vi "sys_integration.vi"() -> ()   [LabVIEW 2016, in "Utilities.lvlib" / "_TEST.lvlib"]
uses:
  _TEST.lvlib
  Drivers/C8855-01/Trigger Mode.ctl
  Drivers/C8855-01/Transfer Mode.ctl
  <vilib>/DAQmx/write.llb/DAQmx Write (Analog 1D DBL 1Chan NSamp).vi
  <vilib>/DAQmx/read.llb/DAQmx Read (Analog 1D DBL 1Chan NSamp).vi
  <vilib>/DAQmx/create/channels.llb/DAQmx Create Channel (AO-Voltage-Basic).vi
  <vilib>/DAQmx/create/channels.llb/DAQmx Create Channel (AI-Voltage-Basic).vi
  <vilib>/DAQmx/create/channels.llb/DAQmx Create Channel (CO-Pulse Generation-Time).vi
  <vilib>/DAQmx/configure/timing.llb/DAQmx Timing (Implicit).vi
  <vilib>/DAQmx/configure/timing.llb/DAQmx Timing (Sample Clock).vi
  <vilib>/DAQmx/configure/trigger.llb/DAQmx Start Trigger (Digital Edge).vi
  <vilib>/DAQmx/miscellaneous.llb/DAQmx Fill In Error Info.vi
  Drivers/C8855-01/C8855-01.lvlib
  <vilib>/measure/NI_MABase.lvlib
  <resource>/objmgr/daqmx.rc
panel:
  in  "Repeats":u16=100
  in  "Offset (V)":dbl format="%0.2p"
  out "Actual Galvo Freq (Hz)":dbl
  in  "Amplitude (V)":dbl=1.0 format="%#_13g"
  out "Sampling Freq (Hz)":dbl
  out "# / Period":i32
  out "Gate Time (s)":dbl
  in  "Galvo Freq (Hz)":u32=100
  in  "Gate Time (us)":u32=100
  out "Data":cluster{dbl[], u16[]}(graph)
  out "Photon Counter ID":u8
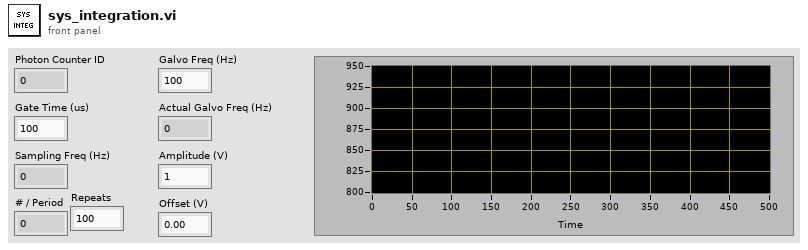
[diagram p1: front panel]
types:
  T1 = typedef "Drivers.lvlib/C8855-01.lvlib/Transfer Mode.ctl" = u8
  T2 = typedef "Drivers.lvlib/C8855-01.lvlib/Trigger Mode.ctl" = u8
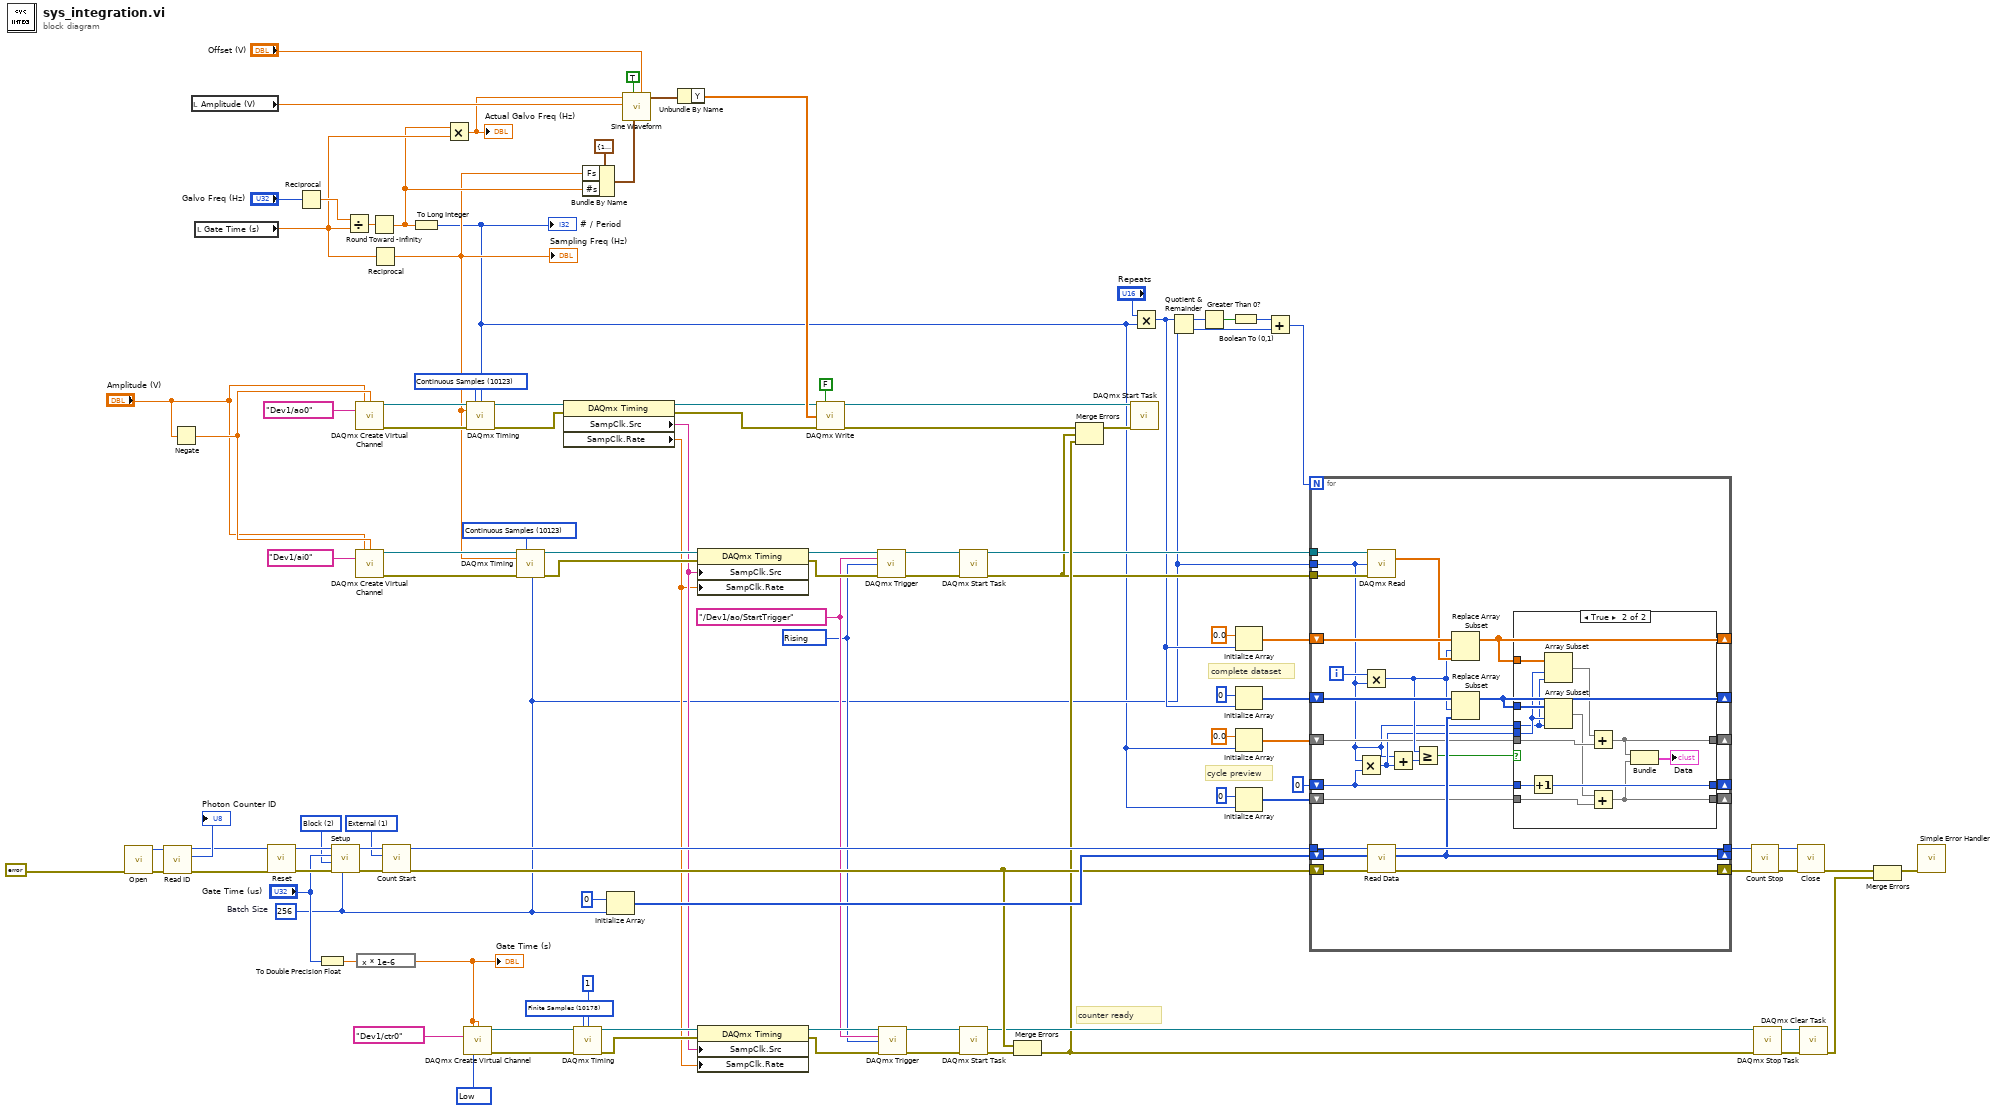
[diagram p0: block diagram]
diagram:
  w32 = 10214 items=["High"=10192, "Low"=10214] ("idle state")
  w28 = 10280 items=["Rising"=10280, "Falling"=10171] ("edge")
  w29 = tag "/Dev1/ao/StartTrigger" ("source")
  w43 = 10123 items=["Finite Samples"=10178, "Continuous Samples"=10123, "Hardware Timed Single Point"=12522] ("sample mode")
  w64 = 10123 items=["Finite Samples"=10178, "Continuous Samples"=10123, "Hardware Timed Single Point"=12522] ("sample mode")
  w78 = T1 2 items=["Single"=1, "Block"=2] ("Transfer Mode")
  w83 = 10178 items=["Finite Samples"=10178, "Continuous Samples"=10123, "Hardware Timed Single Point"=12522] ("sample mode")
  w10 = 256  # Batch Size
  w95 = T2 1 items=["Software", "External"] ("Trigger Mode")
  # "cycle preview"
  # "complete dataset"
  # "counter ready"
  n1 = call "Open.vi"("error in (no error)"=errorcluster {"status"=FALSE, "code"=0, "source"=""}) -> ("error out"=w103:errorcluster, "Handle"=w104:u32)  [unwired: 9 in]
  n2 = call "Read ID.vi"("error in (no error)"=w103, "handle in"=w104) -> ("error out"=w101:errorcluster, "ID"=→"Photon Counter ID":u8, "handle out"=w100:u32)  [unwired: 7 in]
  n3 = Negate(x="Amplitude (V)") -> (-x=w63:dbl)
  n4 = local read "Amplitude (V)"() -> (w59:dbl)
  n5 = local read "Gate Time (s)"() -> (w58:dbl)
  n6 = call "Reset.vi"("error in (no error)"=w101, "handle in"=w100) -> ("error out"=w99:errorcluster, "handle out"=w96:u32)  [unwired: 8 in]
  n7 = Reciprocal(x="Galvo Freq (Hz)") -> (1/x=w67:dbl)
  n8 = To Double Precision Float(number="Gate Time (us)") -> (double precision float=w86:dbl)
  n9 = call "Setup.vi"("Number of Gate"=w10, "error in (no error)"=w99, "Transfer Mode"=w78, "Gate Time (us)"="Gate Time (us)", "Handle"=w96) -> ("error out"=w98:errorcluster, "Handle out"=w97:u32)  [unwired: 5 in]
  n10 = Divide(x=w67, y=w58) -> (x/y=w65:dbl)
  n11 = call-poly <vilib>:"DAQmx Create Virtual Channel.vi"("maximum value"="Amplitude (V)", "minimum value"=w63, "physical channels"=tag "Dev1/ao0") -> ("task out"=w70:refnum<k21>, "error out"=w69:errorcluster)  [unwired: 11 in]
  n12 = call-poly <vilib>:"DAQmx Create Virtual Channel.vi"("maximum value"="Amplitude (V)", "minimum value"=w63, "physical channels"=tag "Dev1/ai0") -> ("task out"=w46:refnum<k21>, "error out"=w45:errorcluster)  [unwired: 11 in]
  n13 = expression code="x * 1e-6"(w86) -> (w66:dbl)
  "Gate Time (s)" <- w66
  n14 = Round Toward -Infinity(1:w65) -> (0:w56:dbl)
  n15 = Reciprocal(x=w58) -> (1/x=w44:dbl)
  "Sampling Freq (Hz)" <- w44
  n16 = call "Count Start.vi"("error in (no error)"=w98, "Trigger Mode"=w95, "handle in"=w97) -> ("error out"=w74:errorcluster, "handle out"=w93:u32)  [unwired: 7 in]
  n17 = To Long Integer(number=w56) -> (32bit integer=w4:i32)
  "# / Period" <- w4
  n18 = Multiply(x=w56, y=w58) -> (x*y=w57:dbl)
  "Actual Galvo Freq (Hz)" <- w57
  n19 = call-poly <vilib>:"DAQmx Create Virtual Channel.vi"("high time"=w66, "low time"=w66, "counter"=tag "Dev1/ctr0" ("physical channels"), "idle state"=w32) -> ("task out"=w85:refnum<k21>, "error out"=w84:errorcluster)  [unwired: 10 in]
  n20 = call-poly <vilib>:"DAQmx Timing.vi"("task/channels in"=w70, "sample mode"=w64, "samples per channel"=w4, "rate"=w44, "error in"=w69) -> ("task out"=w53:refnum<k21>, "error out"=w48:errorcluster)  [unwired: 9 in]
  n21 = call-poly <vilib>:"DAQmx Timing.vi"("task/channels in"=w46, "sample mode"=w43, "samples per channel"=w10, "rate"=w44, "error in"=w45) -> ("task out"=w42:refnum<k21>, "error out"=w40:errorcluster)  [unwired: 9 in]
  n22 = property class="DAQmx Timing"(reference=w53, error in=w48) -> (reference out=w49:refnum<k21>, error out=w47:errorcluster, "SampClk.Src"=w34:tag, "SampClk.Rate"=w33:dbl)
  n23 = call-poly <vilib>:"DAQmx Timing.vi"("task/channels in"=w85, "sample mode"=w83, "samples per channel"=1, "error in"=w84) -> ("task out"=w82:refnum<k21>, "error out"=w35:errorcluster)  [unwired: 10 in]
  n24 = Bundle By Name(cluster=cluster{"Fs":dbl, "#s":dbl} {"Fs"=1000.0, "#s"=1000.0} ("sampling info"), "Fs"=w44, "#s"=w56) -> (w60:cluster{"Fs":dbl, "#s":dbl})
  n25 = Initialize Array(u16 0 ("element"), w10) -> (w92:u16[])
  n26 = call <vilib>:"Sine Waveform.vi"("offset"="Offset (V)", "sampling info"=w60, "reset signal"=TRUE, "amplitude"=w59, "frequency"=w57) -> ("signal out"=w51:waveform(dbl))  [unwired: 5 in, 1 out]
  n27 = Unbundle By Name(w51) -> ("Y"=w50:dbl[])
  n28 = property class="DAQmx Timing"(reference=w42, error in=w40, "SampClk.Src"=w34, "SampClk.Rate"=w33) -> (reference out=w41:refnum<k21>, error out=w39:errorcluster)
  n29 = property class="DAQmx Timing"(reference=w82, error in=w35, "SampClk.Src"=w34, "SampClk.Rate"=w33) -> (reference out=w36:refnum<k21>, error out=w30:errorcluster)
  n30 = call-poly <vilib>:"DAQmx Write.vi"("task/channels in"=w49, "auto start"=FALSE, "data"=w50, "error in"=w47) -> ("task out"=w25:refnum<k21>, "error out"=w24:errorcluster)  [unwired: 9 in, 1 out]
  n31 = call-poly <vilib>:"DAQmx Trigger.vi"("task/channels in"=w41, "source"=w29, "edge"=w28, "error in"=w39) -> ("task out"=w37:refnum<k21>, "error out"=w38:errorcluster)  [unwired: 10 in]
  n32 = call-poly <vilib>:"DAQmx Trigger.vi"("task/channels in"=w36, "source"=w29, "edge"=w28, "error in"=w30) -> ("task out"=w31:refnum<k21>, "error out"=w26:errorcluster)  [unwired: 10 in]
  n33 = call <vilib>:"DAQmx Start Task.vi"("task/channels in"=w37, "error in"=w38) -> ("task out"=w20:refnum<k21>, "error out"=w19:errorcluster)  [unwired: 12 in]
  n34 = call <vilib>:"DAQmx Start Task.vi"("task/channels in"=w31, "error in"=w26) -> ("task out"=w27:refnum<k21>, "error out"=w23:errorcluster)  [unwired: 12 in]
  n35 = Merge Errors(w74, w23) -> (w22:errorcluster)
  n36 = Merge Errors(w24, w19, w22) -> (w21:errorcluster)
  n37 = call <vilib>:"DAQmx Start Task.vi"("task/channels in"=w25, "error in"=w21) -> ()  [unwired: 12 in, 2 out]
  n38 = Multiply(x="Repeats", y=w4) -> (x*y=w12:i32)
  n39 = Quotient & Remainder(x=w12, y=w10) -> (x-y*floor(x/y)=w16:i32, floor(x/y)=w17:i32)
  n40 = Greater Than 0?(x=w16) -> (x > 0?=w15:bool)
  n41 = Boolean To (0,1)(Boolean=w15) -> (0, 1=w14:i16)
  n42 = Initialize Array(0.0 ("element"), w12) -> (w11:dbl[])
  n43 = Initialize Array(u16 0 ("element"), w12) -> (w7:u16[])
  n44 = Initialize Array(0.0 ("element"), w4) -> (w3:dbl[])
  n45 = Initialize Array(u16 0 ("element"), w4) -> (w2:u16[])
  n46 = Add(x=w14, y=w17) -> (x+y=w13:i32)
  n47 = for {
    N: w13 -> [_]
    tunnel: w20 -> [w125]
    tunnel: w19 -> [w124]
    shift-right: [w126] -> w73
    shift-left: w74 -> [w127]
    shift-right: [w119] -> _
    shift-left: w92 -> [w129]
    tunnel: w93 -> [w130]
    tunnel: [w128] -> w91
    shift-right: [w108] -> _
    shift-left: w11 -> [w123]
    tunnel: w10 -> [w106]
    shift-right: [w109] -> _
    shift-left: w7 -> [w120]
    shift-right: [w114] -> _
    shift-left: w3 -> [w115]
    shift-right: [w113] -> _
    shift-left: w2 -> [w112]
    shift-right: [w110] -> _
    shift-left: 0 -> [w111]
    i -> [w121]
    n48 = Multiply(x=w106, y=w111) -> (x*y=w107:i32)
    n49 = Multiply(x=w121, y=w106) -> (x*y=w118:i32)
    n50 = call-poly <vilib>:"DAQmx Read.vi"("task/channels in"=w125, "number of samples per channel"=w106, "error in"=w124) -> ("data"=w122:dbl[])  [unwired: 10 in, 2 out]
    n51 = call "Read Data.vi"("error in (no error)"=w127, "buffer in"=w129, "handle in"=w130) -> ("error out"=w126:errorcluster, "buffer out"=w119:u16[], "handle out"=w128:u32)  [unwired: 6 in]
    n52 = Add(x=w106, y=w107) -> (x+y=w116:i32)
    n53 = Greater Or Equal?(x=w118, y=w116) -> (x >= y?=w117:bool)
    n54 = Replace Array Subset(array=w123, new element=w122, index=w118) -> (w108:dbl[])
    n55 = Replace Array Subset(array=w120, new element=w119, index=w118) -> (w109:u16[])
    n56 = case shown="True" w117 {
      tunnel: w115 -> [w133 w140]
      tunnel: [w133 w136] -> w114
      tunnel: [w132 w134] -> w113
      tunnel: w112 -> [w132 w138]
      tunnel: w111 -> [w131 w142]
      tunnel: [w131 w141] -> w110
      tunnel: w109 -> [_ w146]
      tunnel: w108 -> [_ w145]
      tunnel: w107 -> [_ w144]
      tunnel: w106 -> [_ w143]
      frame False {
      }
      frame True {
        n57 = Increment(x=w142) -> (x+1=w141:i32)
        n58 = Array Subset(array=w145, index=w144, length=w143) -> (w139:dbl[])
        n59 = Array Subset(array=w146, index=w144, length=w143) -> (w137:u16[])
        n60 = Add(x=w139, y=w140) -> (x+y=w136:dbl[])
        n61 = Add(x=w137, y=w138) -> (x+y=w134:u16[])
        n62 = Bundle(w136, w134) -> (→"Data":cluster{dbl[], u16[]})  [unwired: 1 in]
      }
    }
  }
  n63 = call "Count Stop.vi"("error in (no error)"=w73, "handle in"=w91) -> ("error out"=w89:errorcluster, "handle out"=w90:u32)  [unwired: 8 in]
  n64 = call <vilib>:"DAQmx Stop Task.vi"("task/channels in"=w27, "error in"=w22) -> ("task out"=w76:refnum<k21>, "error out"=w77:errorcluster)  [unwired: 12 in]
  n65 = call "Close.vi"("error in (no error)"=w89, "handle in"=w90) -> ("error out"=w81:errorcluster)  [unwired: 9 in]
  n66 = call <vilib>:"DAQmx Clear Task.vi"("task in"=w76, "error in"=w77) -> ("error out"=w79:errorcluster)  [unwired: 13 in]
  n67 = Merge Errors(w81, w79) -> (w80:errorcluster)
  n68 = call <vilib>:"Simple Error Handler.vi"("error in (no error)"=w80) -> ()  [unwired: 4 in, 5 out]
